vi "arrayOfSounds.vi"(11 "Array":string[](array[string])) -> (3 "name or relative path":string)   [LabVIEW 2019]
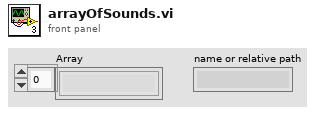
[diagram p1: front panel]
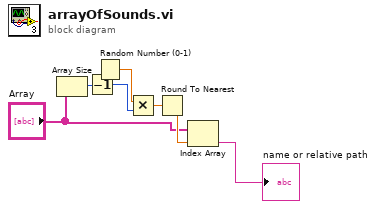
[diagram p0: block diagram]
diagram:
  n1 = Array Size(array="Array") -> (size(s)=w1:i32)
  n2 = Decrement(x=w1) -> (x-1=w2:i32)
  n3 = Random Number (0-1)() -> (number: 0 to 1=w4:dbl)
  n4 = Multiply(x=w4, y=w2) -> (x*y=w5:dbl)
  n5 = Round To Nearest(number=w5) -> (nearest integer value=w6:dbl)
  n6 = Index Array(array="Array", index=w6) -> (element=→"name or relative path":string)
